vi "IMAQ-MWT GALVO Intensity Calibration (HOST).vi"() -> ()   [LabVIEW 2017]
uses:
  Modules/Common/Controls (HOST)/Image Size.ctl
  Modules/Common/Controls (HOST)/REF.ctl
  Modules/Common/Controls (HOST)/Image Queue Bundle.ctl
  Modules/Common/Controls (HOST)/Data to Disk Bundle.ctl
  Modules/Common/Controls (HOST)/File Name Prefix.ctl
  Modules/Common/Controls (HOST)/FPGA REF (MWT).ctl
  Modules/Common/Controls (HOST)/Experiment Mode.ctl
  Modules/Common/Controls (HOST)/Main States.ctl
  Modules/Common/Controls (HOST)/IMAQ Parameters.ctl
  Modules/Common/Controls (HOST)/File REF.ctl
  <vilib>/vision/Avi.llb/IMAQ AVI2 Refnum.ctl
  <vilib>/Utility/error.llb/Error Cluster From Error Code.vi
  <vilib>/rvi/errors/niLvFpgaAdjustHostInterfaceError.vi
  <vilib>/FPGAPlugInAG/Dynamic/niLvFpga_Close_Dynamic.vi
  <vilib>/DAQmx/configure/timing.llb/DAQmx Timing (Sample Clock).vi
  <vilib>/rvi/interface/nirviReadWriteControl/nirviReadWriteControl.xnode
  <vilib>/rvi/interface/nirviCloseFPGA/nirviCloseFPGA.xnode
  NiFpgaLv.dll
  <vilib>/rvi/interface/Simulation/niFpgaSimulationCallBeginRW.vi
  <vilib>/vision/NI_Vision_Development_Module.lvlib
  <vilib>/ptbypt/NI_PtbyPt.lvlib
panel:
  out "Area (Pixels)":dbl[](array[numeric]) format="%#.0f"
  out "Area (Pixels)":dbl format="%#.0f"
  in  "Calibrate":bool
  in  "Stop Button":bool
  out "Scan spots":cluster{"X":i32, "Y":i32}[](array[cluster])=[{"X"=200, "Y"=200}, {"X"=3000, "Y"=200}]
  in  "DAQmx Task Name":refnum<k21>="GALVO"
  out "IR SPOT (Measured)":cluster{"X":i32, "Y":i32}
  in  "Tab Control":enum32{"Setup"}(tab)
  in  "Image Size":T1={"Height"=3072, "Width"=3200}
  in  "Experiment Mode":T2
  in  "Pixel Intensity Range":cluster{"Low":u8, "High":u8}={"Low"=25, "High"=135}
  in  "Exp. Time (S)":dbl=120.0
  in  "Go":bool
  in  "Subtract BG":bool=TRUE
  in  "Replay Interval (ms)":u32=1000
  in  "Swap Bytes":bool
  out "Particle Reports (Pixels)":T3(array[cluster]) {"Orientation" format="%.2f"; "Dimensions"."Height" format="%.2f"; "Dimensions"."Width" format="%.2f"; "Center of Mass"."Y" format="%.2f"; "Center of Mass"."X" format="%.2f"; "Bounding Rect"."Bottom" format="%.2f"; "Bounding Rect"."Right" format="%.2f"; "Bounding Rect"."Top" format="%.2f"; "Bounding Rect"."Left" format="%.2f"; "Number of Holes" format="%.2f"; "Area" format="%.2f"}
  in  "Range":cluster{"Low":sgl, "High":sgl}={"Low"=3.0, "High"=255.0}
  in  "Selection Values":T5(array[cluster])=[{"Measurement Parameter"=18, "Range Lower Value"=50.0, "Range Upper Value"=1000.0, "Range"=FALSE, "Measurement Type"=FALSE}] {"Measurement Parameter" items=["Center of Mass X", "Center of Mass Y", "First Pixel X", "First Pixel Y", "Bounding Rect Left", "Bounding Rect Top", "Bounding Rect Right", "Bounding Rect Bottom", "Max Feret Diameter Start X", "Max Feret Diameter Start Y", "Max Feret Diameter End X", "Max Feret Diameter End Y", "Max Horiz. Segment Length Left", "Max Horiz. Segment Length Right", "Max Horiz. Segment Length Row", "-", "Bounding Rect Width", "Bounding Rect Height", "Bounding Rect Diagonal", "Perimeter", "Convex Hull Perimeter", "Holes' Perimeter", "Max Feret Diameter", "Equivalent Ellipse Major Axis", "Equivalent Ellipse Minor Axis", "Equivalent Ellipse Minor Axis (Feret)", "Equivalent Rect Long Side", "Equivalent Rect Short Side", "Equivalent Rect Diagonal", "Equivalent Rect Short Side (Feret)", "Average Horiz. Segment Length", "Average Vert. Segment Length", "Hydraulic Radius", "Waddel Disk Diameter", "-", "Area", "Holes' Area", "Particle & Holes' Area", "Convex Hull Area", "Image Area", "-", "Number of Holes", "Number of Horiz. Segments", "Number of Vert. Segments", "-", "Orientation", "Max Feret Diameter Orientation", "-", "% Area/Image Area", "% Area/(Particle & Holes' Area)", "Ratio of Equivalent Ellipse Axes", "Ratio of Equivalent Rect Sides", "-", "Elongation Factor", "Compactness Factor", "Heywood Circularity Factor", "Type Factor", "-", "Sum X", "Sum Y", "Sum XX", "Sum XY", "Sum YY", "Sum XXX", "Sum XXY", "Sum XYY", "Sum YYY", "-", "Moment of Inertia XX", "Moment of Inertia XY", "Moment of Inertia YY", "Moment of Inertia XXX", "Moment of Inertia XXY", "Moment of Inertia XYY", "Moment of Inertia YYY", "Norm. Moment of Inertia XX", "Norm. Moment of Inertia XY", "Norm. Moment of Inertia YY", "Norm. Moment of Inertia XXX", "Norm. Moment of Inertia XXY", "Norm. Moment of Inertia XYY", "Norm. Moment of Inertia YYY", "Hu Moment 1", "Hu Moment 2", "Hu Moment 3", "Hu Moment 4", "Hu Moment 5", "Hu Moment 6", "Hu Moment 7"]; "Range Lower Value" format="%.2f"; "Range Upper Value" format="%.2f"}
  out "Number of Particles":i32
  out "Frame #":u32
  out "Frame Rate":u32
  in  "GALVO Input Voltage (V)":T6 {"GALVO 4"."Y" format="%.3f"; "GALVO 4"."X" format="%.3f"; "GALVO 3"."Y" format="%.3f"; "GALVO 3"."X" format="%.3f"; "GALVO 2"."Y" format="%.3f"; "GALVO 2"."X" format="%.3f"; "GALVO 1"."Y" format="%.3f"; "GALVO 1"."X" format="%.3f"}
  in  "Start Location (Pixels)":cluster{"X":i32, "Y":i32}={"X"=300, "Y"=300}
  in  "End Location (Pixels)":cluster{"X":i32, "Y":i32}={"X"=2800, "Y"=2800}
  in  "STEP Size (Pixels)":i32=50
  in  "Y Reverse":bool=TRUE
  in  "X Reverse":bool
  in  "GALVO #":T7(ring)
  out "Elapsed Time (s)":dbl format="%.1f"
  out "Exp. Status":string="Camera Connected"
  out "REF":T8
  out "Command Q":refnum<queue>
  out "Display":T11(plugin-control)
  out "Stopped?":bool
  # "GALVO Intensity Auto Calibration"
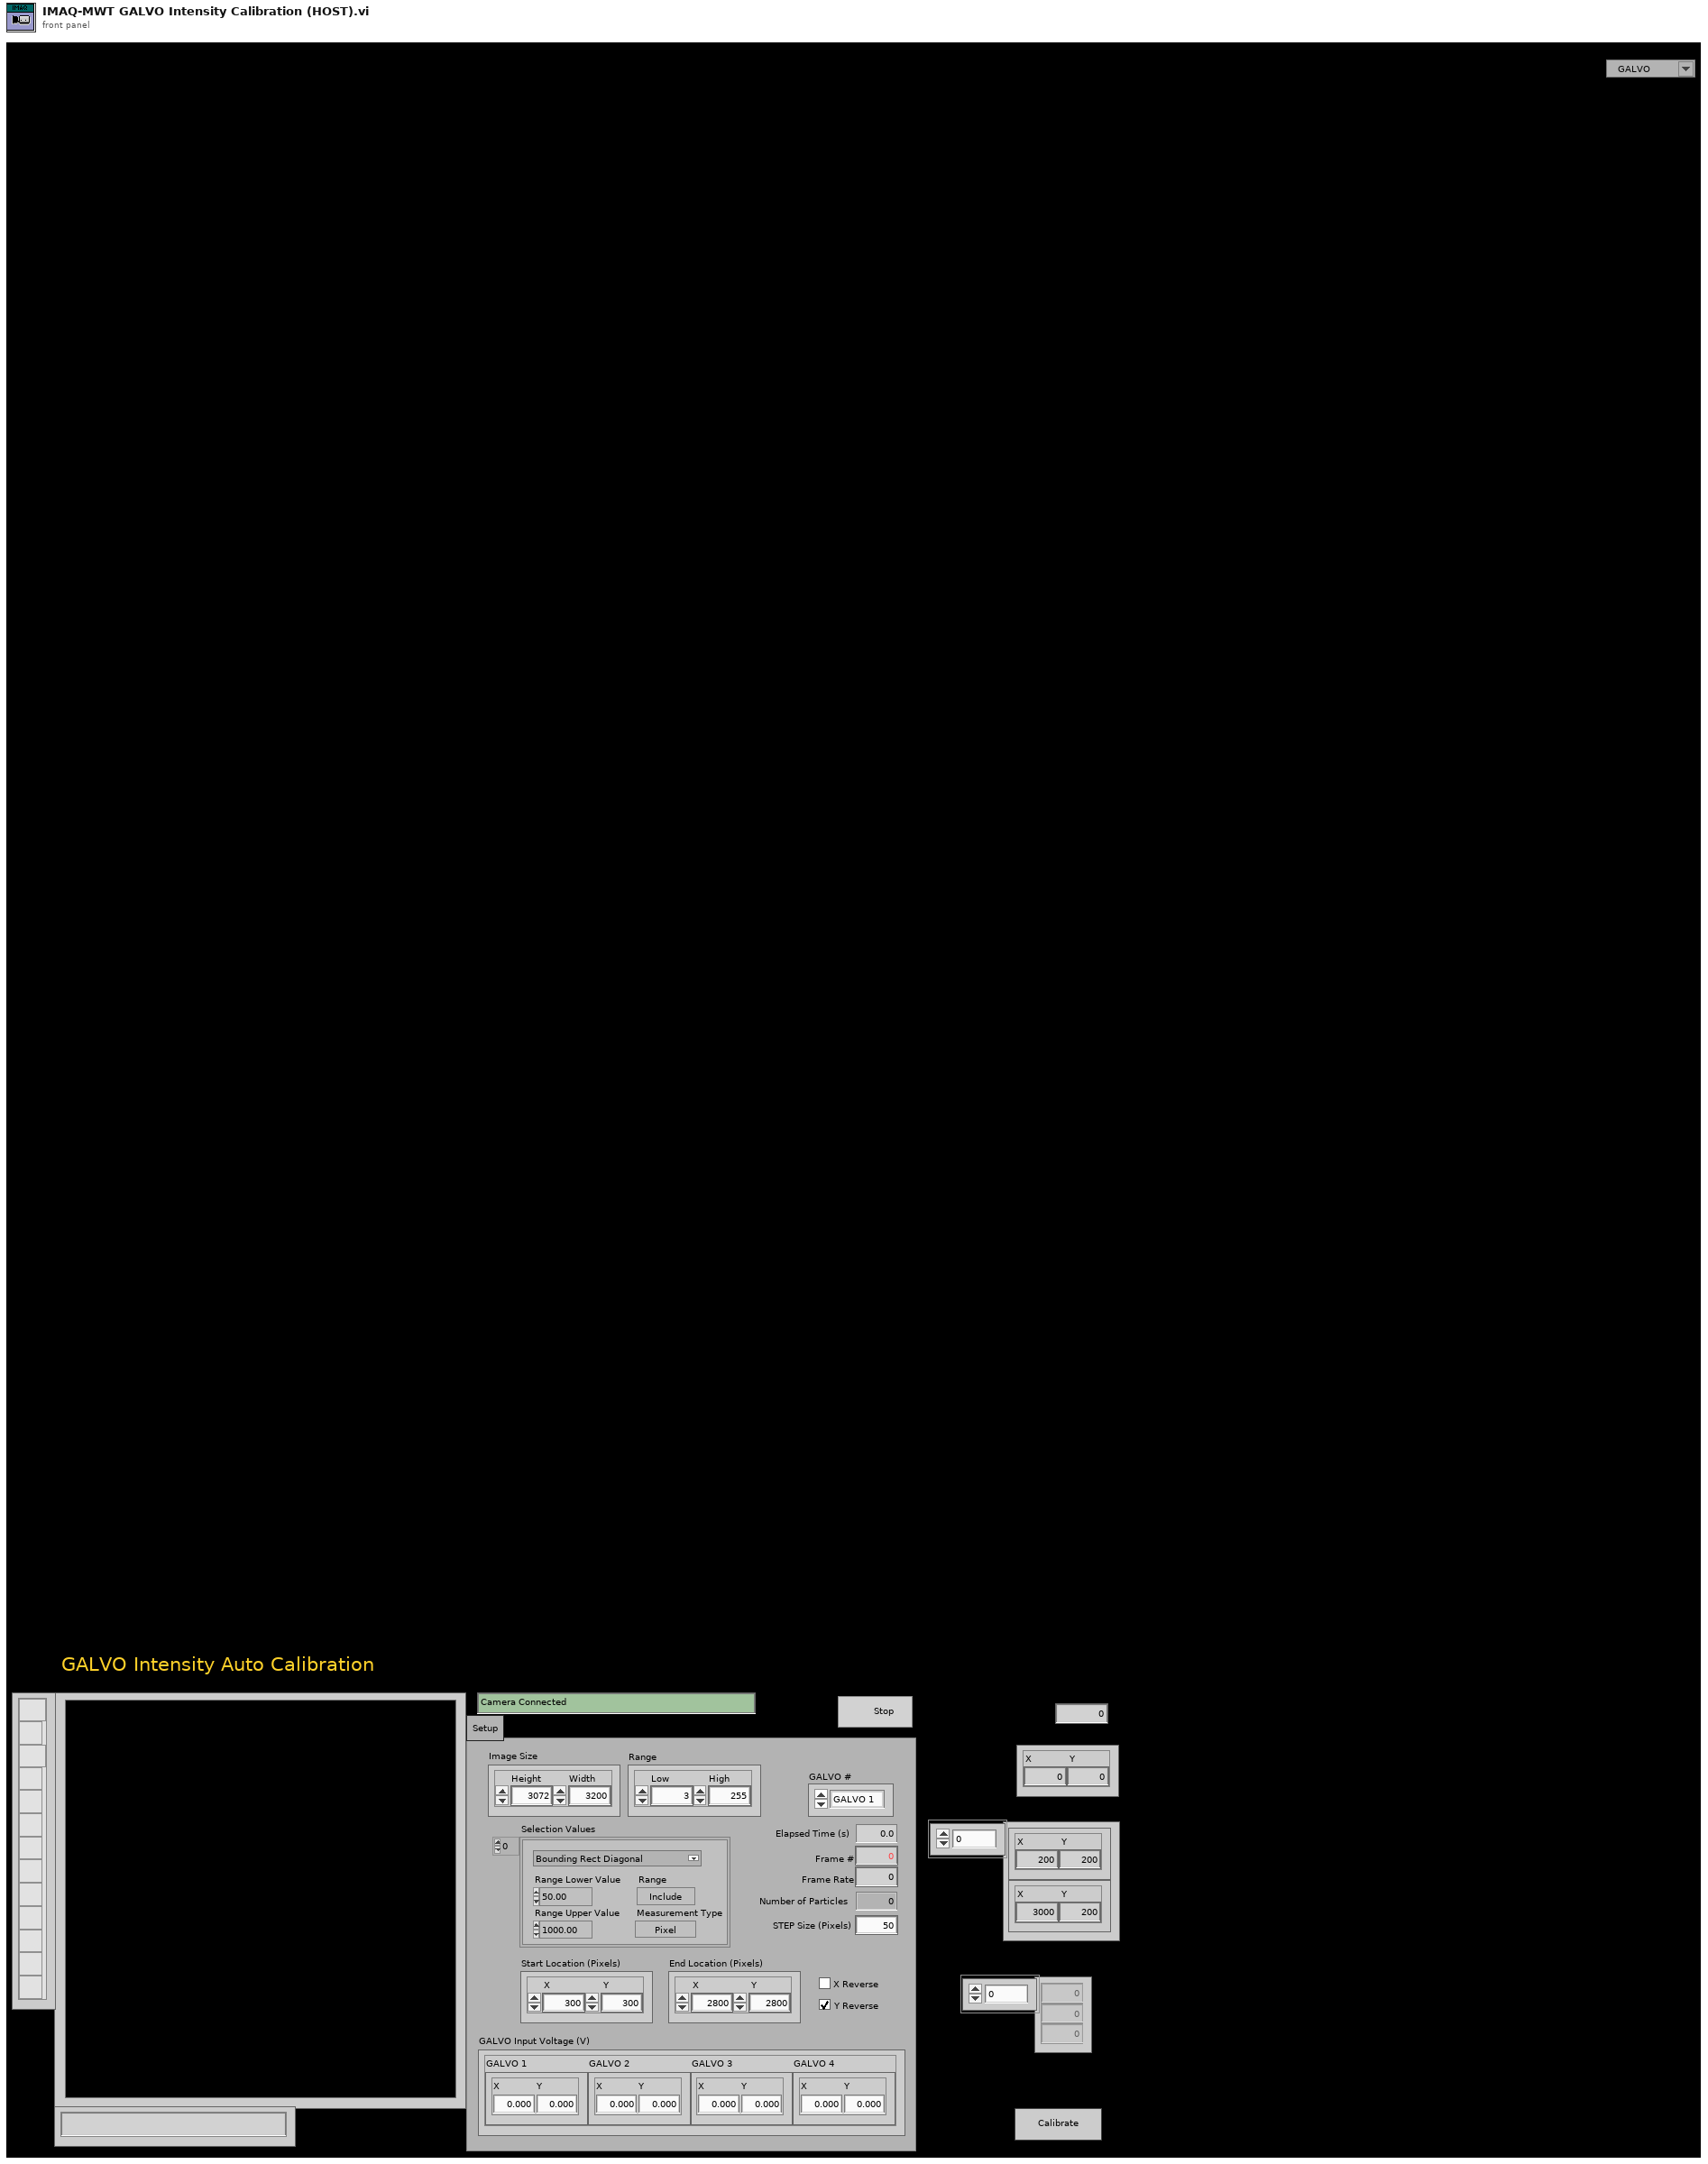
[diagram p1: front panel]
types:
  T1 = typedef "Image Size.ctl" = cluster{"Height":u16, "Width":u16}
  T2 = typedef "Experiment Mode.ctl" = enum16{"Live", "Replay"}
  T3 = cluster{"Area":dbl, "Number of Holes":dbl, "Bounding Rect":cluster{"Left":dbl, "Top":dbl, "Right":dbl, "Bottom":dbl}, "Center of Mass":cluster{"X":dbl, "Y":dbl}, "Orientation":dbl, "Dimensions":cluster{"Width":dbl, "Height":dbl}}[]
  T4 = typedef "Particle Parameters" = i32
  T5 = cluster{"Measurement Parameter":T4, "Range Lower Value":dbl, "Range Upper Value":dbl, "Range":bool, "Measurement Type":bool}[]
  T6 = cluster{"GALVO 1":cluster{"X":dbl, "Y ":dbl}, "GALVO 2":cluster{"X":dbl, "Y ":dbl}, "GALVO 3":cluster{"X":dbl, "Y ":dbl}, "GALVO 4":cluster{"X":dbl, "Y ":dbl}}
  T7 = enum16{"GALVO 1", "GALVO 2", "GALVO 3", "GALVO 4"}
  T8 = typedef "REF.ctl" = cluster{"Queue REF":T9, "FPGA REF (MWT)":T10}
  T9 = typedef "Image Queue Bundle.ctl" = cluster{"Disk Image":refnum<queue>, "Image Blocks":refnum<queue>, "Display Image":refnum<queue>, "BG Image":refnum<queue>, "Tag Image":refnum<queue>, "DLL Input":refnum<queue>, "DMD Input":refnum<queue>, "GALVO Input":refnum<queue>}
  T10 = typedef "FPGA REF (MWT).ctl" = refnum<k20>
  T11 = typedef "IMAQ Image.ctl" = refnum<image>
  T12 = enum8{"Enabled", "Disabled", "Disabled and Grayed Out"}
  T13 = typedef "Main States.ctl" = enum16{"Open FPGA", "Initialize", "Preview", "Acquire Images", "STOP"}
  T14 = typedef "IMAQ Parameters.ctl" = cluster{"File REF":T15, "Frame Data":cluster{"Width":u32, "Height":u32, "Frames Per Second":u32, "Codec":string}, "File Type":string, "Experiment Mode":T2, "Movie File Path":path}
  T15 = typedef "File REF.ctl" = cluster{"AVI REF":T16, "DBDE REF":refnum<file>}
  T16 = typedef "IMAQ AVI2 Refnum.ctl" = refnum<k20>
  T17 = typedef "Data to Disk Bundle.ctl" = cluster{"Frame Number":u64, "Time Stamp (us)":u64, "Image Data":u64[], "Contour":u32[], "Raw Image REF":refnum<data-value>, "Block Image REF":refnum<data-value>, "Block Box":u64[], "SPINE":u32[], "HT Angle":u64[], "Block Position":u64[], "SPINE Count":u32[], "Contour Count":u32[], "SPINE DIR":u8[]}
  T18 = cluster{"Area":dbl, "Number of Holes":dbl, "Bounding Rect":cluster{"Left":dbl, "Top":dbl, "Right":dbl, "Bottom":dbl}, "Center of Mass":cluster{"X":dbl, "Y":dbl}, "Orientation":dbl, "Dimensions":cluster{"Width":dbl, "Height":dbl}}
  T19 = cluster{"Left":dbl, "Top":dbl, "Right":dbl, "Bottom":dbl}
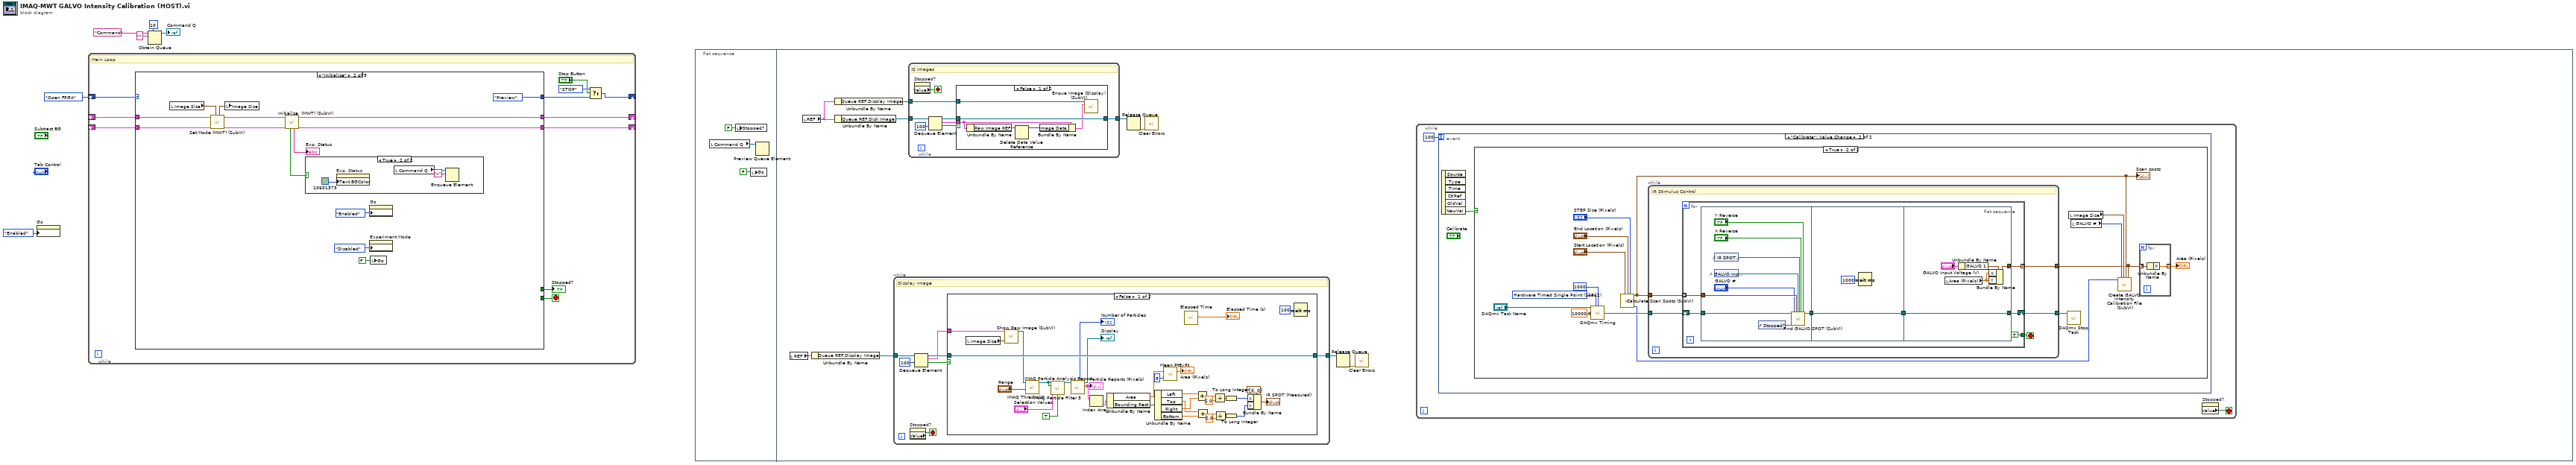
[diagram p0: block diagram]
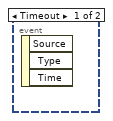
[diagram p2: hidden frame]
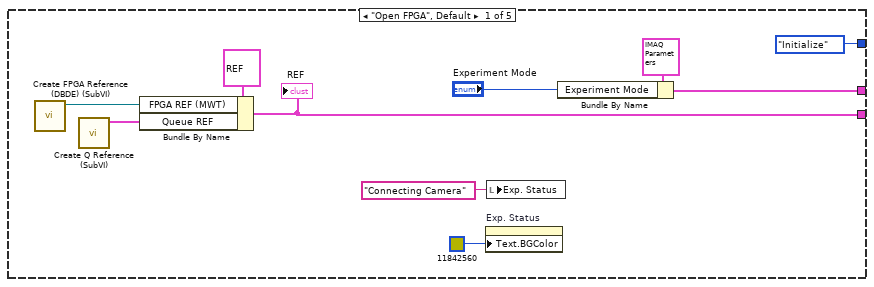
[diagram p6: hidden frame]
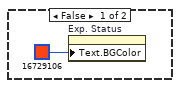
[diagram p7: hidden frame]
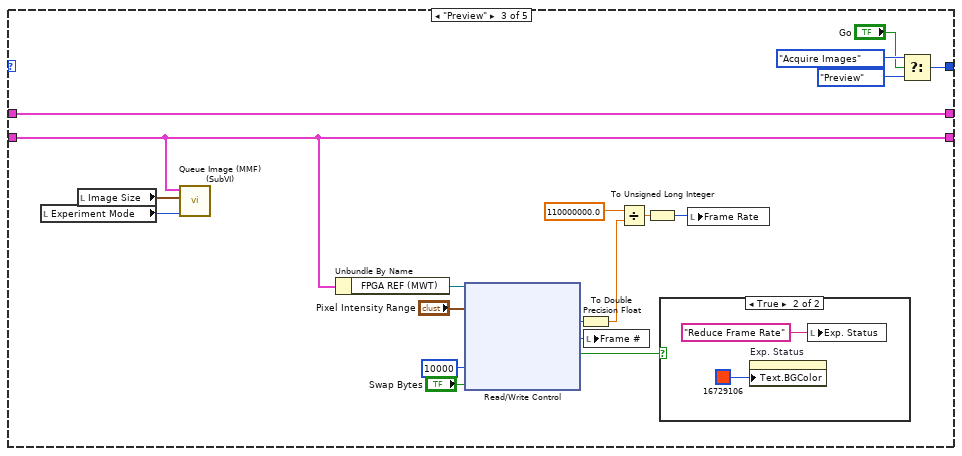
[diagram p8: hidden frame]
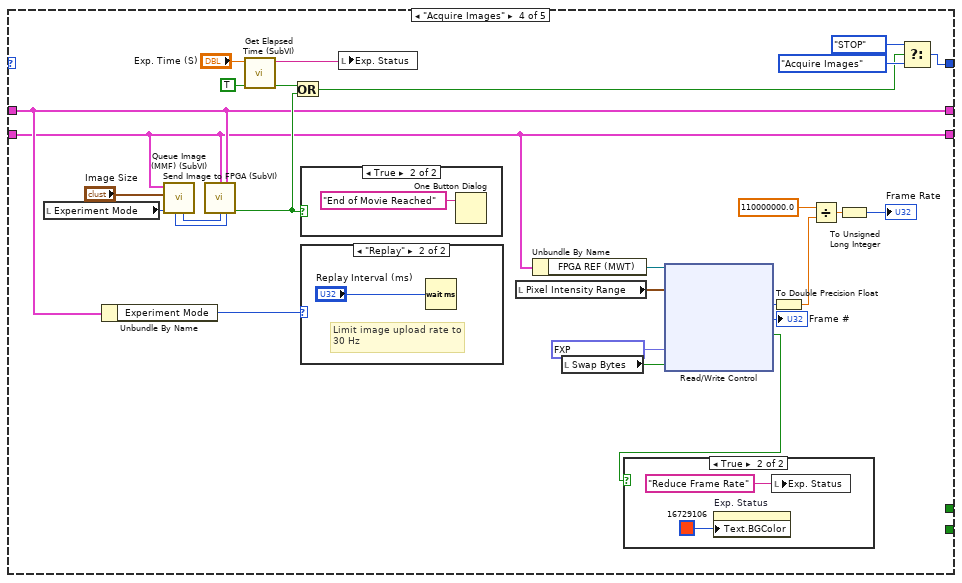
[diagram p10: hidden frame]
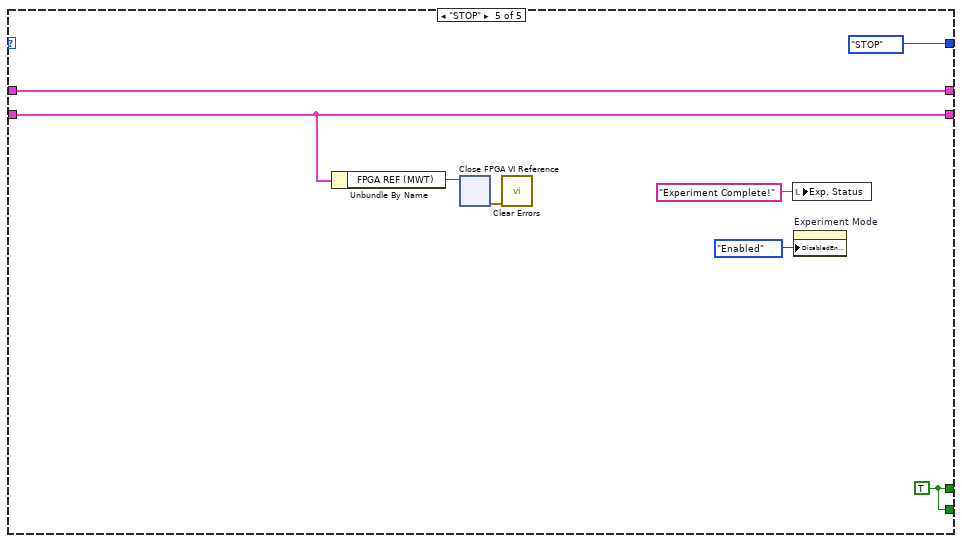
[diagram p14: hidden frame]
diagram:
  n1 = property on="Go" class="Bool (strict)"("DisabledEnum"=T12."Enabled" ("Disabled")) -> ()  [unwired: 2 in, 2 out]
  n2 = while {
    shift-right: [w16] -> _
    shift-left: _ -> [w15]
    shift-right: [w7] -> _
    shift-left: Main_States."Open FPGA" -> [w17]
    shift-right: [w9] -> _
    shift-left: _ -> [w8]
    stop <- w13 stop-if-true
    # "Main Loop"
    n3 = case shown="\"Initialize\"" w17 {
      tunnel: [w24 w28 w49 w72 w102] -> w16
      tunnel: w15 -> [_ w29 w49 w72 w102]
      tunnel: [Main_States."Initialize" Main_States."Preview" w63 w91 Main_States."STOP"] -> w14
      tunnel: [_ _ _ _ w104] -> w13
      tunnel: [_ _ _ _ w104] -> w12
      tunnel: [w18 w33 w56 w75 w101] -> w9
      tunnel: w8 -> [_ w40 w56 w75 w101]
      frame "Open FPGA", Default {
        n4 = call "Create FPGA Reference (DBDE) (SubVI).vi"() -> ("FPGA REF (MWT)"=w26:T10)  [unwired: 11 in]
        n5 = call "Create Q Reference (SubVI).vi"() -> ("Image Queue"=w25:T9)  [unwired: 11 in]
        n6 = Bundle By Name(cluster=T8 {"Queue REF"={"Disk Image"=refnum, "Image Blocks"=refnum, "Display Image"=refnum, "BG Image"=refnum, "Tag Image"=refnum, "DLL Input"=refnum, "DMD Input"=refnum, "GALVO Input"=refnum}, "FPGA REF (MWT)"=refnum}, "FPGA REF (MWT)"=w26, "Queue REF"=w25) -> (w24:T8)
        "REF" <- w24
        n7 = property on="Exp. Status" class="Str"("Text.BGColor"=u32 11842560) -> ()  [unwired: 2 in, 2 out]
        n8 = local write "Exp. Status"("Connecting Camera" ("Exp. Status")) -> ()
        n9 = Bundle By Name(cluster=T14 {"File REF"={"AVI REF"=refnum, "DBDE REF"=refnum}, "Frame Data"={"Width"=0, "Height"=0, "Frames Per Second"=0, "Codec"=""}, "File Type"="", "Experiment Mode"=enum."Live", "Movie File Path"=path "D:/Movies Formatted on November 5th 2015/Clip (2) Formatted.raw"} ("Movie File Property"), "Experiment Mode"="Experiment Mode") -> (w18:T14)
      }
      frame "Initialize" {
        n10 = local read "Image Size"() -> (w31:T1)
        n11 = call "Set Mode (MWT) (SubVI).vi"("Image Size In"=w31, "REF IN"=w29, "Parameters In"=w40) -> ("REF OUT"=w32:T8, "Parameters Out"=w34:T14, "Image Size Out"=w30:T1)  [unwired: 6 in]
        n12 = local write "Image Size"(w30) -> ()
        n13 = call "Initialize  (MWT) (SubVI).vi"("REF IN"=w32, "Parameters In"=w34) -> ("REF OUT"=w28:T8, "Parameters Out"=w33:T14, "Exp. Status"=→"Exp. Status":string, "OK?"=w36:bool)  [unwired: 6 in]
        n14 = case shown="True" w36 {
          frame False {
            n15 = property on="Exp. Status" class="Str"("Text.BGColor"=u32 16729106) -> ()  [unwired: 2 in, 2 out]
          }
          frame True {
            n16 = property on="Exp. Status" class="Str"("Text.BGColor"=u32 10601373) -> ()  [unwired: 2 in, 2 out]
            n17 = local read "Command Q"() -> (w44:refnum<queue>)
            n18 = Enqueue Element(queue=w44, element="v") -> ()  [unwired: 2 in, 3 out]
          }
        }
        n19 = property on="Go" class="Bool (strict)"("DisabledEnum"=T12."Enabled" ("Disabled")) -> ()  [unwired: 2 in, 2 out]
        n20 = property on="Experiment Mode" class="Enum (strict)"("DisabledEnum"=T12."Disabled" ("Disabled")) -> ()  [unwired: 2 in, 2 out]
        n21 = local write "Go"(FALSE ("Go")) -> ()
      }
      frame "Preview" {
        n22 = local read "Experiment Mode"() -> (w47:T2)
        n23 = local read "Image Size"() -> (w53:T1)
        n24 = call "Queue Image (MMF) (SubVI).vi"("Experiment Mode"=w47, "Image Size"=w53, "Data Bundle"=w49) -> ()  [unwired: 9 in]
        n25 = Unbundle By Name(w49) -> ("FPGA REF (MWT)"=w59:T10)
        n26 = xnode "Read/Write Control"("FPGA VI Reference In"=w59, "Pixel Intensity"="Pixel Intensity Range", "Clock Cycles Limit"=u32 10000, "Swap Bytes"="Swap Bytes") -> ("Frame Interval"=w61:u32, "Frame #"=w52:u32, "DMA Timeout"=w51:bool)  [unwired: 1 in, 2 out]
        n27 = To Double Precision Float(number=w61) -> (double precision float=w60:dbl)
        n28 = local write "Frame #"(w52) -> ()
        n29 = Divide(x=110000000.0 ("y"), y=w60) -> (x/y=w57:dbl)
        n30 = To Unsigned Long Integer(number=w57) -> (unsigned 32bit integer=w55:u32)
        n31 = case shown="True" w51 {
          frame False {
          }
          frame True {
            n32 = property on="Exp. Status" class="Str"("Text.BGColor"=u32 16729106) -> ()  [unwired: 2 in, 2 out]
            n33 = local write "Exp. Status"("Reduce Frame Rate" ("Exp. Status")) -> ()
          }
        }
        n34 = local write "Frame Rate"(w55) -> ()
        n35 = Select(t=Main_States."Acquire Images", s="Go", f=Main_States."Preview") -> (s? t:f=w63:T13)
      }
      frame "Acquire Images" {
        n36 = local read "Experiment Mode"() -> (w70:T2)
        n37 = Unbundle By Name(w75) -> ("Experiment Mode"=w74:T2)
        n38 = call "Send Image to FPGA (SubVI).vi"("Data Bundle"=w72, "Parameters"=w75) -> ("TimeStamp"=w69:u64, "Frame Number"=w68:u64, "EOF"=w89:bool)  [unwired: 11 in]
        n39 = call "Queue Image (MMF) (SubVI).vi"("TimeStamp"=w69, "Frame Number"=w68, "Experiment Mode"=w70, "Image Size"="Image Size", "Data Bundle"=w72) -> ()  [unwired: 7 in]
        n40 = call "Get Elapsed Time (SubVI).vi"("Go"=TRUE, "Experiment Time (S)"="Exp. Time (S)") -> ("Done"=w80:bool, "Time Status"=w79:string)  [unwired: 8 in]
        n41 = Or(x=w80, y=w89) -> (x .or. y?=w81:bool)
        n42 = case shown="True" w89 {
          frame False {
          }
          frame True {
            n43 = One Button Dialog(message="End of Movie Reached") -> ()  [unwired: 1 in, 1 out]
          }
        }
        n44 = case shown="\"Replay\"" w74 {
          frame "Live", Default {
          }
          frame "Replay" {
            # "Limit image upload rate to 30 Hz"
            n45 = Wait (ms)(milliseconds to wait="Replay Interval (ms)") -> ()  [unwired: 1 out]
          }
        }
        n46 = local write "Exp. Status"(w79) -> ()
        n47 = local read "Pixel Intensity Range"() -> (w73:cluster{"Low":u8, "High":u8})
        n48 = Unbundle By Name(w72) -> ("FPGA REF (MWT)"=w86:T10)
        n49 = local read "Swap Bytes"() -> (w67:bool)
        n50 = xnode "Read/Write Control"("FPGA VI Reference In"=w86, "Pixel Intensity"=w73, "Significant Angle"=fxp<+,16,3> 0.0699462890625, "Swap Bytes"=w67) -> ("Frame Interval"=w88:u32, "Frame #"=→"Frame #":u32, "DMA Timeout"=w76:bool)  [unwired: 1 in, 2 out]
        n51 = case shown="True" w76 {
          frame False {
          }
          frame True {
            n52 = property on="Exp. Status" class="Str"("Text.BGColor"=u32 16729106) -> ()  [unwired: 2 in, 2 out]
            n53 = local write "Exp. Status"("Reduce Frame Rate" ("Exp. Status")) -> ()
          }
        }
        n54 = To Double Precision Float(number=w88) -> (double precision float=w87:dbl)
        n55 = Divide(x=110000000.0 ("y"), y=w87) -> (x/y=w83:dbl)
        n56 = To Unsigned Long Integer(number=w83) -> (unsigned 32bit integer=→"Frame Rate":u32)
        n57 = Select(t=Main_States."STOP", s=w81, f=Main_States."Acquire Images") -> (s? t:f=w91:T13)
      }
      frame "STOP" {
        w104 = TRUE
        n58 = Unbundle By Name(w102) -> ("FPGA REF (MWT)"=w103:T10)
        n59 = xnode "Close FPGA VI Reference"("FPGA VI Reference In"=w103) -> ("error out"=w98:errorcluster)  [unwired: 1 in]
        n60 = call <vilib>:"Clear Errors.vi"("error in (no error)"=w98) -> ()  [unwired: 5 in, 2 out]
        n61 = local write "Exp. Status"("Experiment Complete!" ("Exp. Status")) -> ()
        n62 = property on="Experiment Mode" class="Enum (strict)"("DisabledEnum"=T12."Enabled" ("Disabled")) -> ()  [unwired: 2 in, 2 out]
      }
    }
    "Stopped?" <- w12
    n63 = Select(t=Main_States."STOP", s="Stop Button", f=w14) -> (s? t:f=w7:T13)
  }
  n64 = Obtain Queue(max queue size (-1, unlimited)=10, name (unnamed)="Command", element data type="" ("name (unnamed)")) -> (queue out=→"Command Q":refnum<queue>)  [unwired: 2 in, 2 out]
  n65 = flat-sequence {
    frame #0 {
      n66 = local read "Command Q"() -> (w108:refnum<queue>)
      n67 = local write "Stopped?"(FALSE ("Stopped?")) -> ()
      n68 = local write "Go"(FALSE ("Go")) -> ()
      n69 = Preview Queue Element(queue=w108) -> ()  [unwired: 2 in, 4 out]
    }
    frame #1 {
      n70 = local read "REF"() -> (w116:T8)
      n71 = local read "REF"() -> (w111:T8)
      n72 = Unbundle By Name(w116) -> ("Queue REF.Display Image"=w115:refnum<queue>)
      n73 = Unbundle By Name(w111) -> ("Queue REF.Display Image"=w112:refnum<queue>)
      n74 = Unbundle By Name(w111) -> ("Queue REF.Disk Image"=w113:refnum<queue>)
      n75 = while {
        tunnel: [w184] -> w117
        tunnel: w115 -> [w183]
        stop <- w181 stop-if-true
        # "Display Image"
        n76 = property on="Stopped?" class="Bool (strict)"() -> ("Value"=w181:bool)  [unwired: 2 in, 2 out]
        n77 = Dequeue Element(queue=w183, timeout in ms (-1)=100) -> (queue out=w185:refnum<queue>, element=w182:T17, timed out?=w186:bool)  [unwired: 1 in, 1 out]
        n78 = case shown="False" w186 {
          tunnel: w185 -> [w220 w221]
          tunnel: [w220 w221] -> w184
          tunnel: w182 -> [w219 _]
          frame False {
            n79 = local read "Image Size"() -> (w217:T1)
            n80 = call "Show Raw Image (SubVI).vi"("Display Data"=w219, "Image Size"=w217) -> ("Image Out"=w216:T11)  [unwired: 17 in]
            n81 = call "IMAQ Threshold"("Range"="Range", "Image Src"=w216) -> ("Image Dst Out"=w215:T11)  [unwired: 8 in, 1 out]
            n82 = call "IMAQ Particle Filter 3"("Image Src"=w215, "Image Dst"=w215, "Selection Values"="Selection Values", "Fill Holes? (F)"=TRUE) -> ("Image Dst Out"=w213:T11)  [unwired: 9 in, 2 out]
            n83 = call "IMAQ Particle Analysis Report"("Image"=w213) -> ("Particle Reports (Pixels)"=w211:T3, "Image Out (duplicate)"=→"Display":T11, "Number of Particles"=→"Number of Particles":i32)  [unwired: 5 in, 3 out]
            "Particle Reports (Pixels)" <- w211
            n84 = Index Array(array=w211) -> (element=w210:T18)  [unwired: 1 in]
            n85 = Unbundle By Name(w210) -> ("Area"=w190:dbl, "Bounding Rect"=w209:T19)
            n86 = Unbundle By Name(w209) -> ("Left"=w208:dbl, "Top"=w201:dbl, "Right"=w207:dbl, "Bottom"=w202:dbl)
            n87 = call <vilib>:"Mean PtByPt.vi"("x"=w190, "sample length"=5) -> ("mean"=→"Area (Pixels)":dbl)  [unwired: 2 in, 1 out]
            n88 = call "Elapsed Time"() -> ("Elapsed Time (s)"=→"Elapsed Time (s)":dbl)  [unwired: 12 in, 7 out]
            n89 = Add(x=w208, y=w207) -> (x+y=w206:dbl)
            n90 = Add(x=w201, y=w202) -> (x+y=w203:dbl)
            n91 = Divide(x=w206, y=2.0) -> (x/y=w200:dbl)
            n92 = Divide(x=w203, y=2.0) -> (x/y=w199:dbl)
            n93 = To Long Integer(number=w200) -> (32bit integer=w195:i32)
            n94 = To Long Integer(number=w199) -> (32bit integer=w194:i32)
            n95 = Bundle By Name(cluster=cluster{"X":i32, "Y":i32} {"X"=0, "Y"=0}, "X"=w195, "Y"=w194) -> (→"IR SPOT (Measured)":cluster{"X":i32, "Y":i32})
            n96 = Wait (ms)(milliseconds to wait=u32 100) -> ()  [unwired: 1 out]
          }
          frame True {
          }
        }
      }
      n97 = while {
        tunnel: [w172] -> w114
        tunnel: w113 -> [w166]
        tunnel: w112 -> [w171]
        stop <- w167 stop-if-true
        # "Q Images"
        n98 = property on="Stopped?" class="Bool (strict)"() -> ("Value"=w167:bool)  [unwired: 2 in, 2 out]
        n99 = Dequeue Element(queue=w166, timeout in ms (-1)=100) -> (queue out=w169:refnum<queue>, element=w170:T17, timed out?=w168:bool)  [unwired: 1 in, 1 out]
        n100 = case shown="False" w168 {
          tunnel: w169 -> [w179 w180]
          tunnel: [w179 w180] -> w172
          tunnel: w171 -> [w178 _]
          tunnel: w170 -> [w176 _]
          frame False {
            n101 = Unbundle By Name(w176) -> ("Raw Image REF"=w177:refnum<data-value>)
            n102 = Delete Data Value Reference(data value reference=w177) -> (data value=w175:u64[])  [unwired: 1 in, 1 out]
            n103 = Bundle By Name(cluster=w176, "Image Data"=w175) -> (w174:T17)
            n104 = call "Enque Image (Display) (SubVI).vi"("Data Bundle"=w174, "Display Image REF"=w178) -> ()  [unwired: 10 in]
          }
          frame True {
          }
        }
      }
      n105 = Release Queue(queue=w114) -> (error out=w109:errorcluster)  [unwired: 2 in, 2 out]
      n106 = call <vilib>:"Clear Errors.vi"("error in (no error)"=w109) -> ()  [unwired: 5 in, 2 out]
      n107 = Release Queue(queue=w117) -> (error out=w110:errorcluster)  [unwired: 2 in, 2 out]
      n108 = call <vilib>:"Clear Errors.vi"("error in (no error)"=w110) -> ()  [unwired: 5 in, 2 out]
      n109 = while {
        stop <- w119 stop-if-true
        n110 = event shown="[1] \"Calibrate\": Value Change" {
          selector: _ -> [_ _]
          dyn-events: _ -> [_ _]
          timeout: 100 -> [_ _]
          event Timeout {
            n111 = event-data() -> ()  [unwired: 1 in, 3 out]
          }
          event "Calibrate": Value Change {
            n112 = event-data() -> ("NewVal"=w120:bool)  [unwired: 1 in, 5 out]
            n113 = case shown="True" w120 {
              frame False {
              }
              frame True {
                w133 = 12522 items=["Finite Samples"=10178, "Continuous Samples"=10123, "Hardware Timed Single Point"=12522] ("sample mode")
                n114 = call-poly <vilib>:"DAQmx Timing.vi"("task/channels in"="DAQmx Task Name", "sample mode"=w133, "samples per channel"=1000, "rate"=10000.0) -> ("task out"=w132:refnum<k21>)  [unwired: 10 in, 1 out]
                n115 = call "Calculate Scan Spots (SubVI).vi"("Start Location (Pixels)"="Start Location (Pixels)", "End Location (Pixels)"="End Location (Pixels)", "STEP Size (Pixels)"="STEP Size (Pixels)") -> ("Scan Spots (Array)"=w124:cluster{"X":i32, "Y":i32}[], "Spot Count"=w123:i32[])  [unwired: 11 in]
                "Scan spots" <- w124
                n116 = while {
                  tunnel: [w142] -> w130
                  tunnel: w132 -> [w141]
                  tunnel: w124 -> [w139]
                  tunnel: [w138] -> w122
                  stop <- w140 stop-if-true
                  # "IR Stimulus Control"
                  n117 = for {
                    tunnel: w139 -> [w147] mode=indexing
                    shift-right: [w149] -> w142
                    shift-left: w141 -> [w148]
                    tunnel: [TRUE ("Stopped?")] -> w140
                    tunnel: [w145] -> w138 mode=indexing
                    n118 = flat-sequence {
                      tunnel: w148 -> [w157]
                      tunnel: w147 -> [w156]
                      tunnel: [w158] -> w144
                      tunnel: w144 -> [w160]
                      tunnel: [w160] -> w143
                      tunnel: [w165] -> w149
                      tunnel: w143 -> [w165]
                      tunnel: [w162] -> w145
                      frame #0 {
                        n119 = control-ref of="IR SPOT (Measured)"() -> (w155:refnum<vi>)
                        n120 = control-ref of="GALVO Input Voltage (V)"() -> (w154:refnum<vi>)
                        n121 = control-ref of="Stopped?"() -> (w150:refnum<vi>)
                        n122 = call "Find GALVO SPOT (SubVI).vi"("REF In"=w157, "Stopped?"=w150, "GALVO #"="GALVO #", "IR SPOT (Target)"=w156, "GALVO Input Voltage (V)"=w154, "IR SPOT (Measured)"=w155, "X Reverse"="X Reverse", "Y Reverse"="Y Reverse") -> ("REF Out"=w158:refnum<k21>)  [unwired: 19 in]
                      }
                      frame #1 {
                        n123 = Wait (ms)(milliseconds to wait=u32 1000) -> ()  [unwired: 1 out]
                      }
                      frame #2 {
                        n124 = local read "Area (Pixels)"() -> (w161:dbl)
                        n125 = Unbundle By Name("GALVO Input Voltage (V)") -> ("GALVO 1"=w163:cluster{"X":dbl, "Y ":dbl})
                        n126 = Bundle By Name(cluster=w163, "X"=w161, "Y"=w161) -> (w162:cluster{"X":dbl, "Y ":dbl})
                      }
                    }
                  }
                }
                n127 = call <vilib>:"DAQmx Stop Task.vi"("task/channels in"=w130) -> ()  [unwired: 13 in, 2 out]
                n128 = local read "Image Size"() -> (w126:T1)
                n129 = local read "GALVO #"() -> (w125:T7)
                n130 = call "Create GALVO Intensity Calibration File (SubVI).vi"("Spot Count"=w123, "GALVO #"=w125, "Image Size"=w126, "Scan Spots (Array)"=w124, "GALVO Voltage Inputs"=w122) -> ()  [unwired: 15 in]
                n131 = for {
                  tunnel: w122 -> [w137] mode=indexing
                  tunnel: [w136] -> w121 mode=indexing
                  n132 = Unbundle By Name(w137) -> ("X"=w136:dbl)
                }
                "Area (Pixels)" <- w121
              }
            }
          }
        }
        n133 = property on="Stopped?" class="Bool (strict)"() -> ("Value"=w119:bool)  [unwired: 2 in, 2 out]
      }
    }
  }
